vi "StartPostPurge.vi"(10 "t":string, 11 "Operate":bool) -> (3 "f":string)   [LabVIEW 2015]
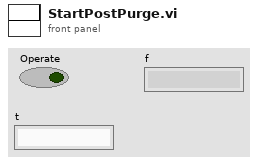
[diagram p1: front panel]
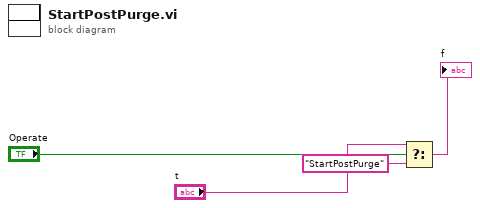
[diagram p0: block diagram]
diagram:
  n1 = Select(t="t", s="Operate", f="StartPostPurge") -> (s? t:f=→"f":string)
